vi "setCommandString.vi"(5 "addTab? (F)":bool, 6 "addLF_onlyIfNeeded? (T)":bool=TRUE, 7 "addLF? (T)":bool=TRUE, 8 "addTimeAndChevron? (T)":bool=TRUE, 9 "numLines":i32=50, 10 "stringToAdd":string, 11 "UI Data In":T1={"controlTabState"=[], "pathToSTLFiles"=path "", "availableObjs"=[], "objectNames"=[], "addedObjs"=[], "selectedObj"={"Name"="", "objectFiles"=[], "center"={"X"=0.0, "Y"=0.0, "Z"=0.0}, "extent"={"X"=0.0, "Y"=0.0, "Z"=0.0}, "allowedMotion"=enum."XY", "mountOn"=enum."yArm", "Movements"=[], "extraInfo"=[], "hasPOI?"=FALSE, "POI"={"X"=0.0, "Y"=0.0, "Z"=0.0}, "posOffset"={"X"=0.0, "Y"=0.0, "Z"=0.0}, "referenceNum"=refnum}, "3DPictureObjRef"=refnum, "yPOI_Home"={"X"=0.0, "Y"=0.0, "Z"=0.0}, "yPOI_Current"={"X"=0.0, "Y"=0.0, "Z"=0.0}, "yPOI_Added?"=FALSE, "homePos_Offset"={"X"=0.0, "Y"=0.0, "Z"=0.0}, "breadBoardOriginOffset"={"X"=0.0, "Y"=0.0, "Z"=0.0}, "XYtranslateObjControls"=[], "ZtranslateObjControls"=[], "pBot_controls"=[], "pBot_VISA"="", "commandLog"="", "pBotConnected?"=FALSE, "pBot_currentEEPROMsettings"="", "realTimeInfoControls"=[], "pBot_tempSensor1"=0.0, "pBot_tempSensor2"=0.0, "realTimeInfoTextColor"=[], "disconnectPBot_Event"=refnum, "needToHomeY?"=FALSE, "pBot_relativePositioning"=FALSE, "pBot_minPos"={"X"=0.0, "Y"=0.0, "Z"=0.0}, "pBot_maxPos"={"X"=0.0, "Y"=0.0, "Z"=0.0}, "pBot_homeOffset"={"X"=0.0, "Y"=0.0, "Z"=0.0}, "textColorGreen"=9174826, "textColorRed"=16750216, "textColorGray"=9868950, "transVisualizationControls"=[], "needToHomeXY?"=FALSE, "pBot_minScanRegion"={"X"=0.0, "Y"=0.0, "Z"=0.0}, "pBot_maxScanRegion"={"X"=0.0, "Y"=0.0, "Z"=0.0}, "pBot_scanN"={"X"=0, "Y"=0, "Z"=0}, "connectedInstruments"=[], "isScanning?"=FALSE, "Wavelengths"=[], "usb2000p_controlRefs"=[]}) -> (0 "error out":errorcluster, 2 "UI Data Out":T1={"controlTabState"=[], "pathToSTLFiles"=path "", "availableObjs"=[], "objectNames"=[], "addedObjs"=[], "selectedObj"={"Name"="", "objectFiles"=[], "center"={"X"=0.0, "Y"=0.0, "Z"=0.0}, "extent"={"X"=0.0, "Y"=0.0, "Z"=0.0}, "allowedMotion"=enum."XY", "mountOn"=enum."yArm", "Movements"=[], "extraInfo"=[], "hasPOI?"=FALSE, "POI"={"X"=0.0, "Y"=0.0, "Z"=0.0}, "posOffset"={"X"=0.0, "Y"=0.0, "Z"=0.0}, "referenceNum"=refnum}, "3DPictureObjRef"=refnum, "yPOI_Home"={"X"=0.0, "Y"=0.0, "Z"=0.0}, "yPOI_Current"={"X"=0.0, "Y"=0.0, "Z"=0.0}, "yPOI_Added?"=FALSE, "homePos_Offset"={"X"=0.0, "Y"=0.0, "Z"=0.0}, "breadBoardOriginOffset"={"X"=25.4, "Y"=12.7, "Z"=12.7}, "XYtranslateObjControls"=[], "ZtranslateObjControls"=[], "pBot_controls"=[], "pBot_VISA"="", "commandLog"="", "pBotConnected?"=FALSE, "pBot_currentEEPROMsettings"="", "realTimeInfoControls"=[], "pBot_tempSensor1"=0.0, "pBot_tempSensor2"=0.0, "realTimeInfoTextColor"=[], "disconnectPBot_Event"=refnum, "needToHomeY?"=FALSE, "pBot_relativePositioning"=FALSE, "pBot_minPos"={"X"=0.0, "Y"=0.0, "Z"=0.0}, "pBot_maxPos"={"X"=0.0, "Y"=0.0, "Z"=0.0}, "pBot_homeOffset"={"X"=0.0, "Y"=0.0, "Z"=0.0}, "textColorGreen"=9174826, "textColorRed"=16750216, "textColorGray"=9868950, "transVisualizationControls"=[], "needToHomeXY?"=FALSE, "pBot_minScanRegion"={"X"=0.0, "Y"=0.0, "Z"=0.0}, "pBot_maxScanRegion"={"X"=0.0, "Y"=0.0, "Z"=0.0}, "pBot_scanN"={"X"=0, "Y"=0, "Z"=0}, "connectedInstruments"=[], "isScanning?"=FALSE, "Wavelengths"=[], "usb2000p_controlRefs"=[]}, 3 "outputCommandString":string)   [LabVIEW 2015]
uses:
  controls/UI Data.ctl
  processedObjectInfo.ctl
  controls/scanInstrumentInfo.ctl
panel:
  # "this error is not used for anything!\nIt is just to control the flow better\nin the calling VI!"
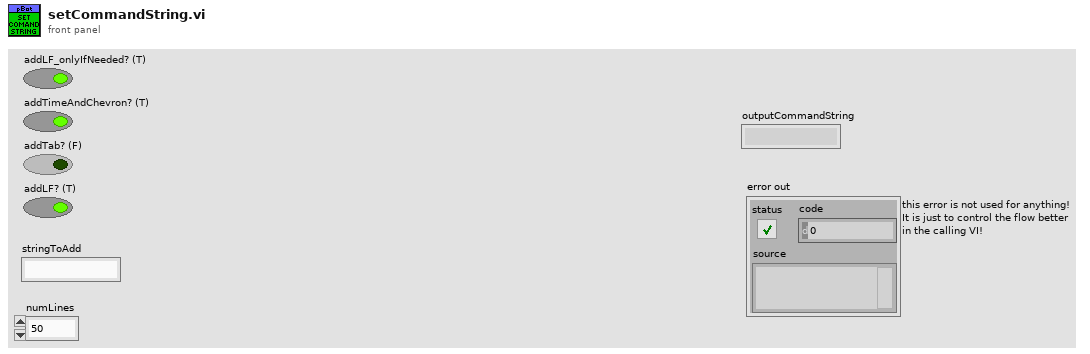
[diagram p1: front panel]
types:
  T1 = typedef "UI Data.ctl" = cluster{"controlTabState":bool[], "pathToSTLFiles":path, "availableObjs":T2[], "objectNames":string[], "addedObjs":T2[], "selectedObj":T2, "3DPictureObjRef":refnum<vi>, "yPOI_Home":cluster{"X":dbl, "Y":dbl, "Z":dbl}, "yPOI_Current":cluster{"X":dbl, "Y":dbl, "Z":dbl}, "yPOI_Added?":bool, "homePos_Offset":cluster{"X":dbl, "Y":dbl, "Z":dbl}, "breadBoardOriginOffset":cluster{"X":dbl, "Y":dbl, "Z":dbl}, "XYtranslateObjControls":refnum<vi>[], "ZtranslateObjControls":refnum<vi>[], "pBot_controls":refnum<vi>[], "pBot_VISA":refnum<visa-resource-name>, "commandLog":string, "pBotConnected?":bool, "pBot_currentEEPROMsettings":string, "realTimeInfoControls":refnum<vi>[], "pBot_tempSensor1":dbl, "pBot_tempSensor2":dbl, "realTimeInfoTextColor":u32[], "disconnectPBot_Event":refnum<user-event>, "needToHomeY?":bool, "pBot_relativePositioning":bool, "pBot_minPos":cluster{"X":dbl, "Y":dbl, "Z":dbl}, "pBot_maxPos":cluster{"X":dbl, "Y":dbl, "Z":dbl}, "pBot_homeOffset":cluster{"X":dbl, "Y":dbl, "Z":dbl}, "textColorGreen":u32, "textColorRed":u32, "textColorGray":u32, "transVisualizationControls":refnum<vi>[], "needToHomeXY?":bool, "pBot_minScanRegion":cluster{"X":sgl, "Y":sgl, "Z":sgl}, "pBot_maxScanRegion":cluster{"X":sgl, "Y":sgl, "Z":sgl}, "pBot_scanN":cluster{"X":u16, "Y":u16, "Z":u16}, "connectedInstruments":T3[], "isScanning?":bool, "Wavelengths":dbl[], "usb2000p_controlRefs":refnum<vi>[]}
  T2 = typedef "processedObjectInfo.ctl" = cluster{"Name":string, "objectFiles":cluster{"Location":path, "Color":cluster{"R":dbl, "G":dbl, "B":dbl, "A":dbl}}[], "center":cluster{"X":dbl, "Y":dbl, "Z":dbl}, "extent":cluster{"X":dbl, "Y":dbl, "Z":dbl}, "allowedMotion":enum16{"XY", "Z"}, "mountOn":enum16{"yArm", "breadBoard"}, "Movements":cluster{"Type":enum16{"rr", "ra", "tr", "ta"}, "vector":cluster{"X":dbl, "Y":dbl, "Z":dbl}, "scalar":dbl}[], "extraInfo":cluster{"parameter":string, "dataType":string, "vector":cluster{"X":dbl, "Y":dbl, "Z":dbl}, "scalar":dbl}[], "hasPOI?":bool, "POI":cluster{"X":dbl, "Y":dbl, "Z":dbl}, "posOffset":cluster{"X":dbl, "Y":dbl, "Z":dbl}, "referenceNum":refnum<vi>}
  T3 = typedef "scanInstrumentInfo.ctl" = cluster{"Name":string, "VISAname":refnum<visa-resource-name>, "1D_dataArraySize":u16, "extraInfo":variant, "error":errorcluster}
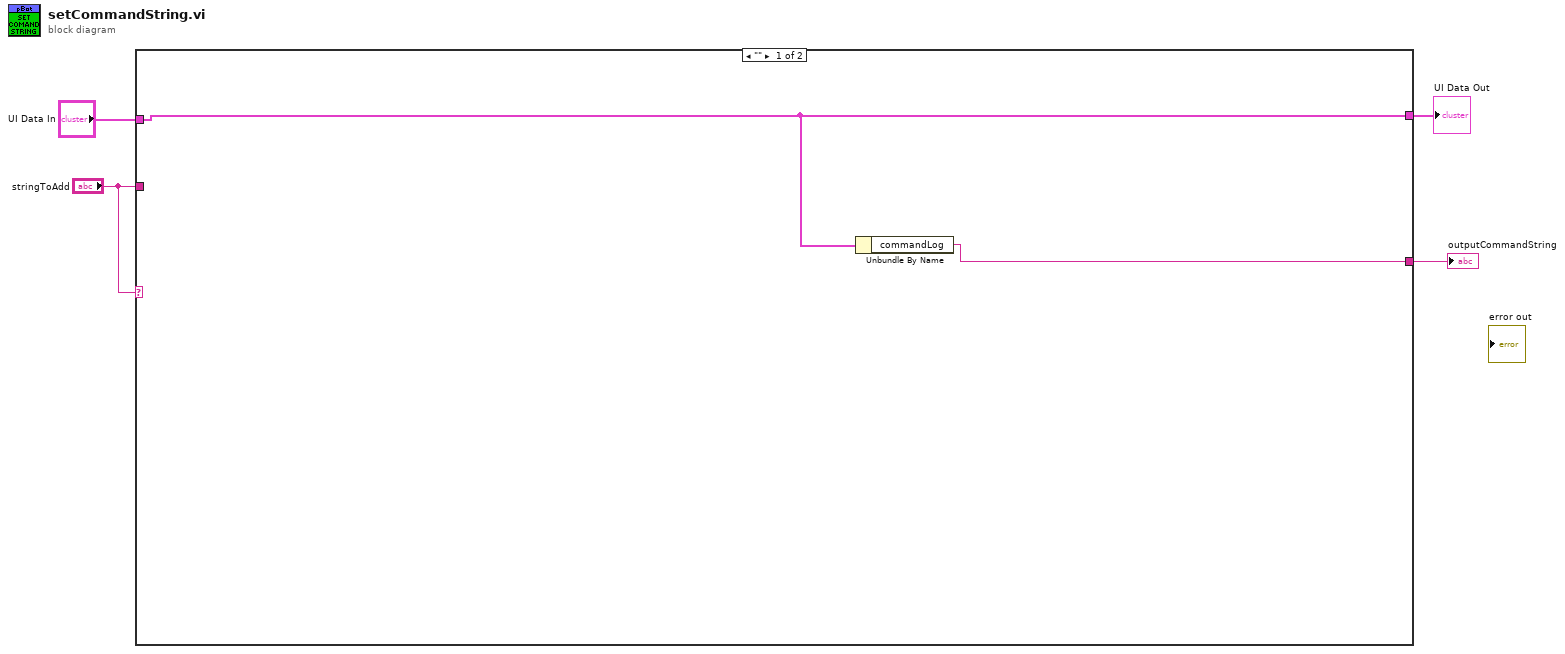
[diagram p0: block diagram]
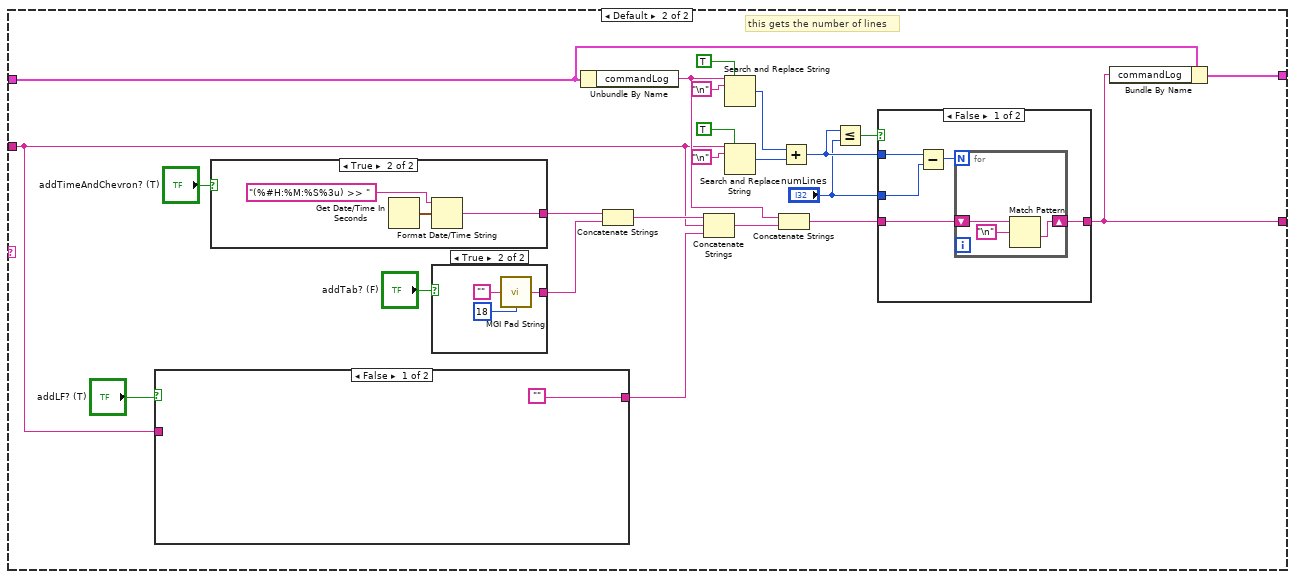
[diagram p2: hidden frame]
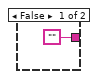
[diagram p3: hidden frame]
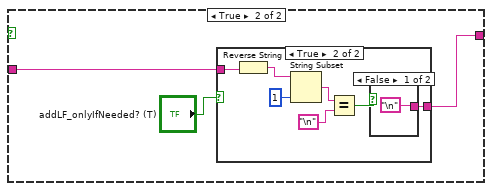
[diagram p4: hidden frame]
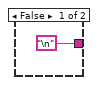
[diagram p5: hidden frame]
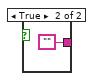
[diagram p6: hidden frame]
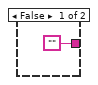
[diagram p7: hidden frame]
diagram:
  n1 = case shown="\"\"" "stringToAdd" {
    tunnel: "stringToAdd" -> [_ w8]
    tunnel: "UI Data In" -> [w6 w14]
    tunnel: [w6 w13] -> w3
    tunnel: [w5 w7] -> w1
    frame "" {
      n2 = Unbundle By Name(w6) -> ("commandLog"=w5:string)
    }
    frame Default {
      # "this gets the number of lines"
      n3 = case shown="False" "addLF? (T)" {
        tunnel: ["" w35] -> w16
        tunnel: w8 -> [_ w36]
        frame False {
        }
        frame True {
          n4 = case shown="True" "addLF_onlyIfNeeded? (T)" {
            tunnel: w36 -> [_ w45]
            tunnel: ["\n" w39] -> w35
            frame False {
            }
            frame True {
              n5 = Reverse String(1:w45) -> (0:w44:string)
              n6 = String Subset(string=w44, length (rest)=1 ("length (rest)")) -> (substring=w42:string)  [unwired: 1 in]
              n7 = Equal?(x=w42, y="\n") -> (x = y?=w40:bool)
              n8 = case shown="False" w40 {
                tunnel: ["\n" ""] -> w39
                frame False {
                }
                frame True {
                }
              }
            }
          }
        }
      }
      n9 = case shown="True" "addTimeAndChevron? (T)" {
        tunnel: ["" w49] -> w11
        frame False {
        }
        frame True {
          n10 = Get Date/Time In Seconds() -> (seconds since 1Jan1904=w50:timestamp)
          n11 = Format Date/Time String(time format string (%c)="(%#H:%M:%S%3u) >> ", seconds (now)=w50) -> (date/time string=w49:string)  [unwired: 1 in]
        }
      }
      n12 = case shown="True" "addTab? (F)" {
        tunnel: ["" w31] -> w10
        frame False {
        }
        frame True {
          n13 = call <userlib>:"MGI Pad String.vi"("String In"="", "End Length"=u32 18) -> ("String Out"=w31:string)  [unwired: 13 in]
        }
      }
      n14 = Unbundle By Name(w14) -> ("commandLog"=w15:string)
      n15 = Concatenate Strings(w11, w10) -> (w9:string)
      n16 = Concatenate Strings(w9, w8, w16) -> (w19:string)
      n17 = Search and Replace String(replace all?=TRUE ("replace all? (F)"), input string=w15, search string="\n") -> (number of replacements=w25:i32)  [unwired: 5 in, 3 out]
      n18 = Search and Replace String(replace all?=TRUE ("replace all? (F)"), input string=w8, search string="\n") -> (number of replacements=w24:i32)  [unwired: 5 in, 3 out]
      n19 = Concatenate Strings(w15, w19) -> (w22:string)
      n20 = Add(x=w25, y=w24) -> (x+y=w21:i32)
      n21 = Less Or Equal?(x=w21, y="numLines") -> (x <= y?=w23:bool)
      n22 = case shown="False" w23 {
        tunnel: [w52 w60] -> w7
        tunnel: w22 -> [w53 w60]
        tunnel: w21 -> [w56 _]
        tunnel: "numLines" -> [w55 _]
        frame False {
          n23 = Subtract(x=w56, y=w55) -> (x-y=w54:i32)
          n24 = for {
            N: w54 -> [_]
            shift-right: [w57] -> w52
            shift-left: w53 -> [w59]
            n25 = Match Pattern(string=w59, regular expression="\n") -> (after substring=w57:string)  [unwired: 1 in, 3 out]
          }
        }
        frame True {
        }
      }
      n26 = Bundle By Name(cluster=w14, "commandLog"=w7) -> (w13:T1)
    }
  }
  "UI Data Out" <- w3
  "outputCommandString" <- w1
